vi "RSZVB Trace Add Diagram Area.vi"(6 "Channel (1)":i32=1, 7 "Trace Name (Trc1)":string="Trc1", 8 "error in (no error)":errorcluster {"code" format="%.0x"}, 9 "Window (Trace) (1)":i32=1, 10 "Window (1)":i32=1, 11 "VISA session":refnum<visa-resource-name>) -> (0 "error out":errorcluster {"code" format="%.0x"}, 3 "dup VISA session":refnum<visa-resource-name>)   [LabVIEW 2011]
doc: "This VI creates a new trace in a new diagram area and assigns the trace to the selected channel. The new trace is created with the default trace and channel settings. \n\nRemote-control command(s):\nCALCulate<Ch>:PARameter:SDEFine '<string>', 'S21'\nDISPlay:WINDow<Wnd>:STATe ON\nDISPlay:WINDow<Wnd>:TRACe<WndTr>:FEED <string>"
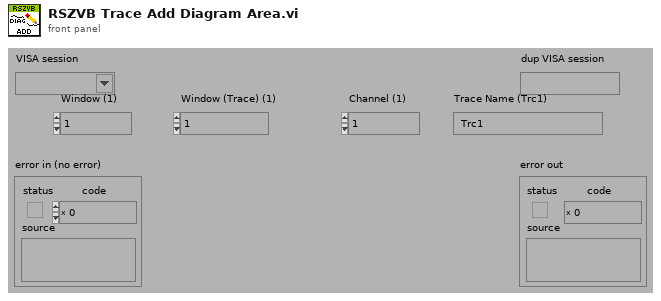
[diagram p1: front panel]
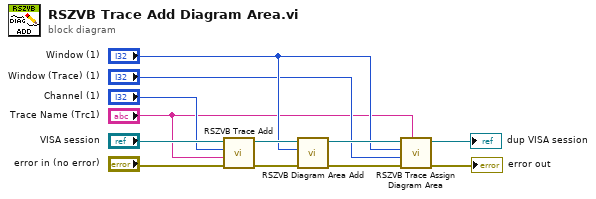
[diagram p0: block diagram]
diagram:
  n1 = call "RSZVB Trace Add.vi"("error in (no error)"="error in (no error)", "Trace Name (Trc1)"="Trace Name (Trc1)", "Channel (1)"="Channel (1)", "VISA session"="VISA session") -> ("error out"=w10:errorcluster, "dup VISA session"=w9:refnum<visa-resource-name>)  [unwired: 6 in]
  n2 = call "RSZVB Diagram Area Add.vi"("error in (no error)"=w10, "Window (1)"="Window (1)", "VISA session"=w9) -> ("error out"=w7:errorcluster, "dup VISA session"=w6:refnum<visa-resource-name>)  [unwired: 7 in]
  n3 = call "RSZVB Trace Assign Diagram Area.vi"("Trace Name (Trc1)"="Trace Name (Trc1)", "error in (no error)"=w7, "Window (Trace) (1)"="Window (Trace) (1)", "Window (1)"="Window (1)", "VISA session"=w6) -> ("error out"=→"error out":errorcluster, "dup VISA session"=→"dup VISA session":refnum<visa-resource-name>)  [unwired: 5 in]
